vi "Main Read Processed Incoming Messages.vi"(8 "error in":errorcluster, 11 "internal data":T1={"J1939 XNET Settings"={"XNET Database"="", "XNET Cluster"="", "CAN port"="", "Baud rate [Bd]"=0, "J1939 Network Address"=0, "Name"=0, "Termination"=0}, "j1939 queues"={"Processed Outgoing"=refnum, "Process Outgoing"=refnum, "stop notifier"=refnum, "error queue"=refnum, "active dtc"=refnum, "processed inc"=refnum}, "fgv references"={"BAM Buffer"=refnum, "CM Buffer"=refnum, "CM Gen"=refnum, "BAM Gen"=refnum, "Address Claims"=refnum, "RQST"=refnum, "scaling lut"=refnum, "data lut"=refnum, "cyclic scheduler"=refnum}, "frame in"="", "frame out"="", "timing"={"tb to j1939 queue timeout"=100, "j1939 to tb queue timeout"=100, "dtc loop period (ms)"=100, "CAN in loop period (ms)"=100, "process incoming queue timeout (ms)"=100, "Outgoing Write Decimation"=0, "process outgoing loop rate (ms)"=0, "periodic outgoing queue timeout (ms)"=10, "CAN out queue timeout (ms)"=100}}) -> ()   [LabVIEW 2013, in "J1939.lvlib"]
uses:
  J1939.lvlib
  API Types/Internal Data.ctl
  API Types/XNET Settings.ctl
  API Types/Setup Information Cluster.ctl
  API Types/CAN Outgoing Message Cluster.ctl
  API Types/Convert DTCs Cluster.ctl
  <vilib>/xnet/xnet.llb/XNET Frame CAN.ctl
  <vilib>/xnet/xnet.llb/XNET Frame Type CAN.ctl
  TP/TP List References.ctl
  BAM/BAM Buffer Connections List_Ref.ctl
  Connection Mode/Connection Mode Generation Connection Ref.ctl
  BAM/BAM Generation Connections List_Ref.ctl
  LUTs/J1939 Address Table Reference.ctl
  RQST/RQST Lookup Table Reference.ctl
  LUTs/J1939 Conversion Lookup Table Reference.ctl
  LUTs/J1939 Data Lookup Table Reference.ctl
  LUTs/Cyclic Frame Scheduler Lut Reference.ctl
  Configuration/TypeDefs/timing configuration.ctl
  <vilib>/xnet/xnet.llb/XNET Convert (Frame Raw to Signal).vi
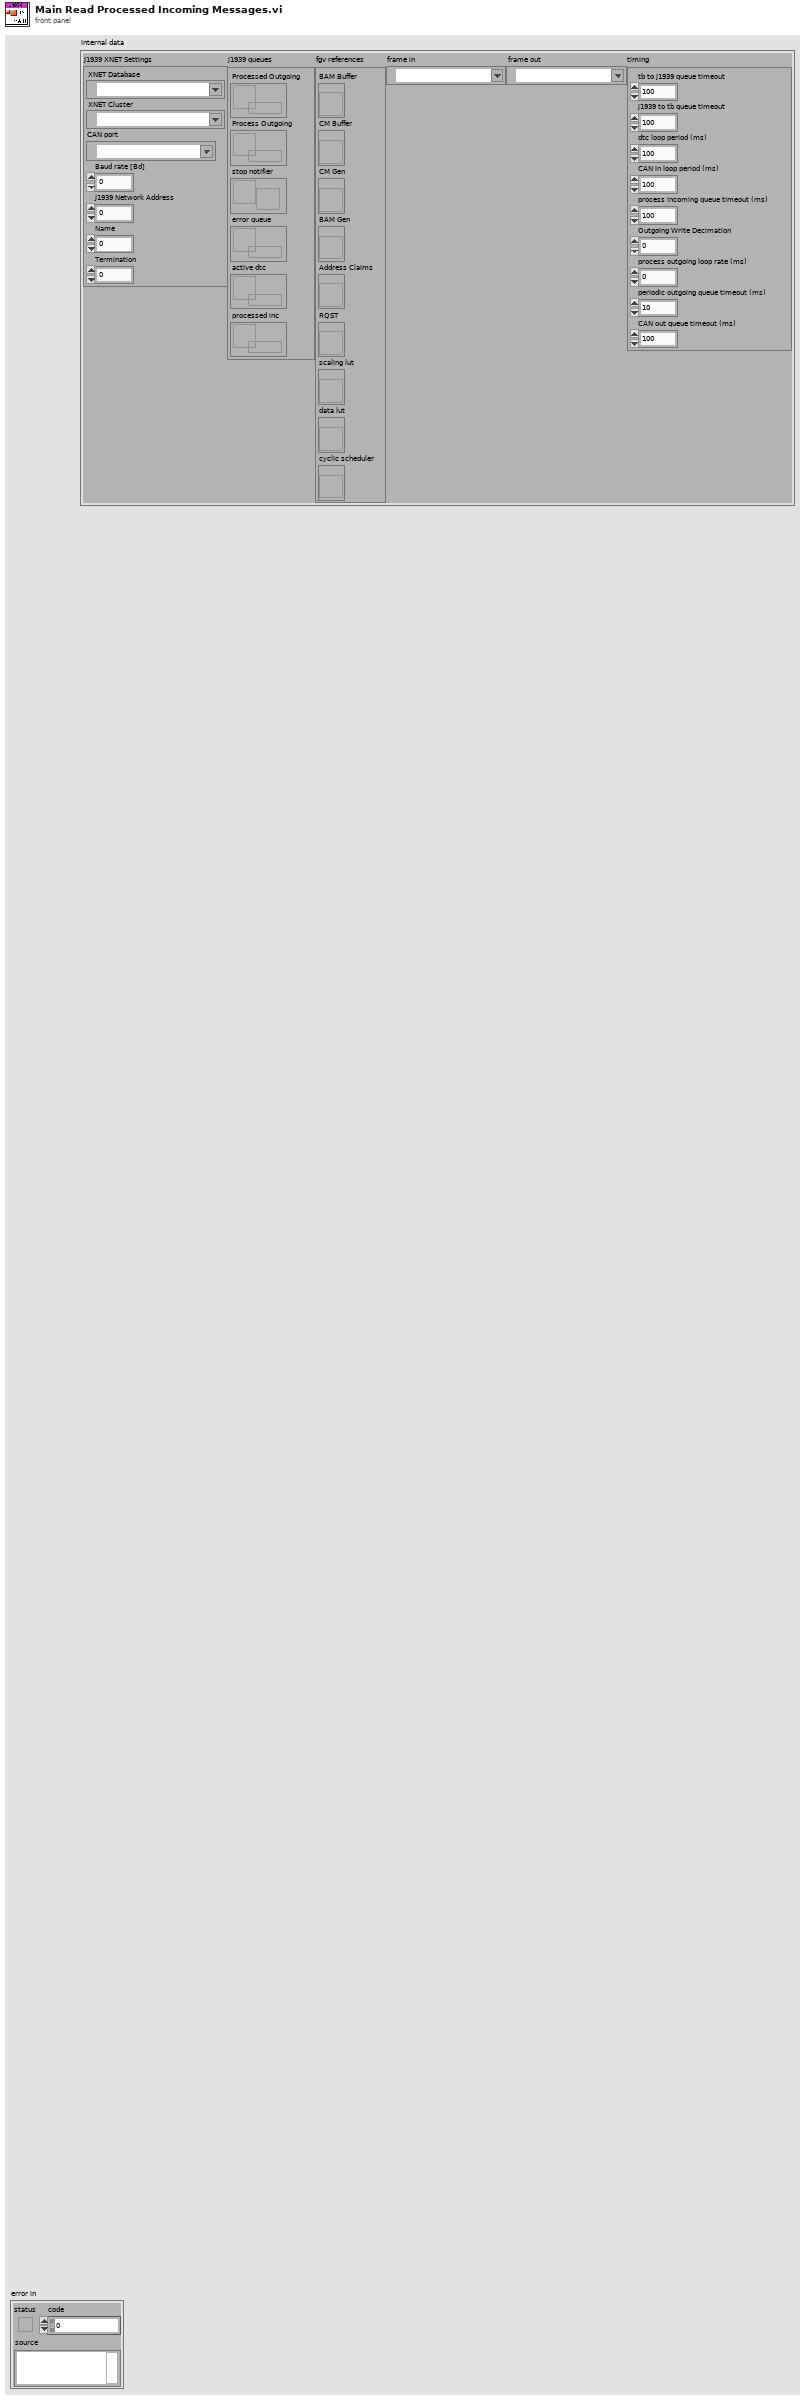
[diagram p1: front panel]
types:
  T1 = typedef "J1939.lvlib/Internal Data.ctl" = cluster{"J1939 XNET Settings":T2, "j1939 queues":T3, "fgv references":T4, "frame in":refnum<k21>, "frame out":refnum<k21>, "timing":T13}
  T2 = typedef "J1939.lvlib/XNET settings.ctl" = cluster{"XNET Database":refnum<k21>, "XNET Cluster":refnum<k21>, "CAN port":refnum<k21>, "Baud rate [Bd]":u32, "J1939 Network Address":u8, "Name":u64, "Termination":u32}
  T3 = typedef "J1939.lvlib/Setup Information Cluster.ctl" = cluster{"Processed Outgoing":refnum<queue>, "Process Outgoing":refnum<queue>, "stop notifier":refnum<notifier>, "error queue":refnum<queue>, "active dtc":refnum<queue>, "processed inc":refnum<queue>}
  T4 = typedef "J1939.lvlib/TP List References.ctl" = cluster{"BAM Buffer":T5, "CM Buffer":T5, "CM Gen":T6, "BAM Gen":T7, "Address Claims":T8, "RQST":T9, "scaling lut":T10, "data lut":T11, "cyclic scheduler":T12}
  T5 = typedef "J1939.lvlib/BAM Buffer Connections List_Ref.ctl" = refnum<vi>
  T6 = typedef "J1939.lvlib/Connection Mode Generation Connection Ref.ctl" = refnum<vi>
  T7 = typedef "J1939.lvlib/BAM Generation Connections List_Ref.ctl" = refnum<vi>
  T8 = typedef "J1939.lvlib/J1939 Address Table Reference.ctl" = refnum<vi>
  T9 = typedef "J1939.lvlib/RQST Lookup Table Reference.ctl" = refnum<vi>
  T10 = typedef "J1939.lvlib/J1939 Conversion Lookup Table Reference.ctl" = refnum<vi>
  T11 = typedef "J1939.lvlib/J1939 Data Lookup Table Reference.ctl" = refnum<vi>
  T12 = typedef "J1939.lvlib/cyclic frame scheduler lut reference.ctl" = refnum<vi>
  T13 = typedef "J1939.lvlib/timing configuration.ctl" = cluster{"tb to j1939 queue timeout":i32, "j1939 to tb queue timeout":i32, "dtc loop period (ms)":i32, "CAN in loop period (ms)":i32, "process incoming queue timeout (ms)":i32, "Outgoing Write Decimation":u32, "process outgoing loop rate (ms)":i32, "periodic outgoing queue timeout (ms)":i32, "CAN out queue timeout (ms)":i32}
  T14 = typedef "XNET Frame CAN.ctl" = cluster{"timestamp":timestamp, "payload":u8[], "identifier":u32, "type":T15, "extended?":bool, "echo?":bool}
  T15 = typedef "XNET Frame Type CAN.ctl" = u8
  T16 = typedef "J1939.lvlib/J1939 Conversion Lookup Table Parameters Cluster.ctl" = cluster{"Conversion":refnum<k21>, "Array Position":cluster{"Offset":u32, "Length":u32}, "Length":u32, "Conv ID":u32}
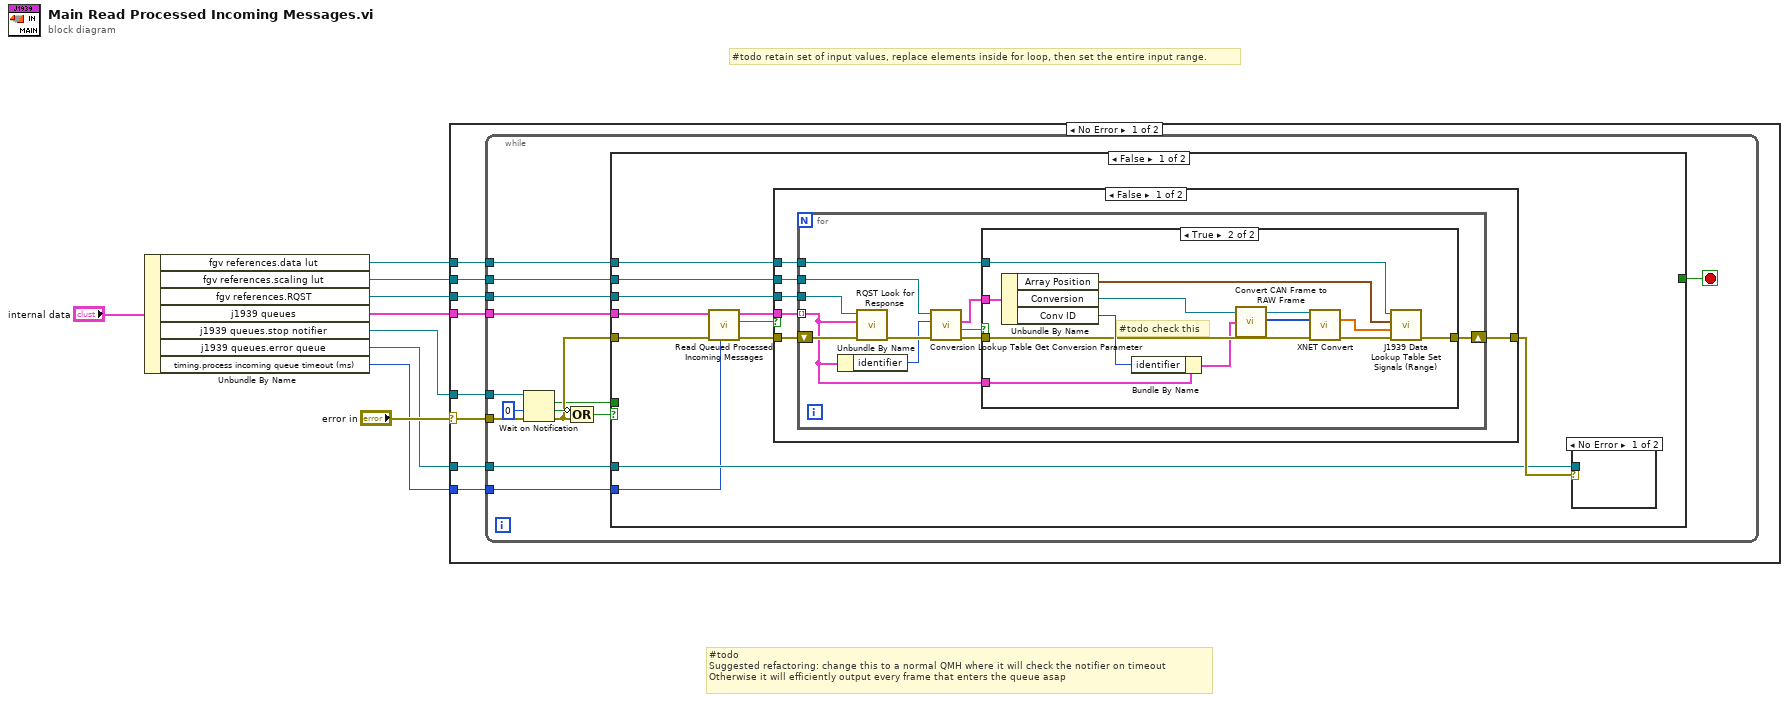
[diagram p0: block diagram]
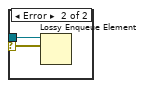
[diagram p2: hidden frame]
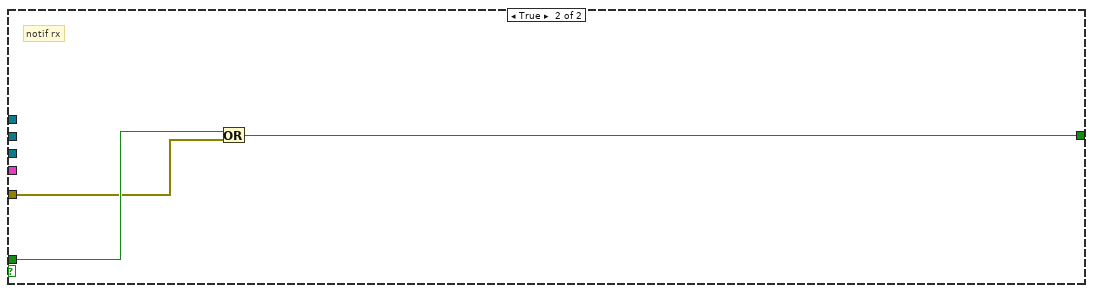
[diagram p5: hidden frame]
diagram:
  # "#todo retain set of input values, replace elements inside for loop, then set the entire input range."
  # "#todo\nSuggested refactoring: change this to a normal QMH where it will check the notifier on timeout\nOtherwise it will efficiently output every frame that enters the queue asap"
  n1 = Unbundle By Name("internal data") -> ("fgv references.data lut"=w4:T11, "fgv references.scaling lut"=w5:T10, "fgv references.RQST"=w6:T9, "j1939 queues"=w7:T3, "j1939 queues.stop notifier"=w3:refnum<notifier>, "j1939 queues.error queue"=w2:refnum<queue>, "timing.process incoming queue timeout (ms)"=w1:i32)
  n2 = case shown="No Error" "error in" {
    selector: "error in" -> [w17 _]
    tunnel: w3 -> [w16 _]
    tunnel: w7 -> [w15 _]
    tunnel: w6 -> [w14 _]
    tunnel: w5 -> [w13 _]
    tunnel: w4 -> [w12 _]
    tunnel: w2 -> [w11 _]
    tunnel: w1 -> [w10 _]
    frame No Error {
      n3 = while {
        tunnel: w16 -> [w19]
        tunnel: w17 -> [w31]
        tunnel: w15 -> [w25]
        tunnel: w14 -> [w24]
        tunnel: w13 -> [w23]
        tunnel: w12 -> [w22]
        tunnel: w11 -> [w20]
        tunnel: w10 -> [w18]
        stop <- w26 stop-if-true
        n4 = Wait on Notification(notifier=w19, timeout in ms (-1)=0, error in (no error)=w31) -> (notification=w27:bool, timed out?=w30:bool, error out=w28:errorcluster)  [unwired: 1 in, 1 out]
        n5 = Compound Arithmetic op=OR(invert w30, w28) -> (w29:bool)
        n6 = case shown="False" w29 {
          tunnel: w28 -> [w39 w76]
          tunnel: w27 -> [_ w78]
          tunnel: [_ w77] -> w26
          tunnel: w25 -> [w38 _]
          tunnel: w24 -> [w37 _]
          tunnel: w23 -> [w36 _]
          tunnel: w22 -> [w35 _]
          tunnel: w20 -> [w33 _]
          tunnel: w18 -> [w32 _]
          frame False {
            n7 = call "Read Queued Processed Incoming Messages.vi"("timeout in ms (-1)"=w32, "error in"=w39, "j1939 queues"=w38) -> ("error out"=w42:errorcluster, "timed out?"=w40:bool, "Frames"=w41:T14[])  [unwired: 6 in]
            n8 = case shown="False" w40 {
              tunnel: w36 -> [w50 _]
              tunnel: w35 -> [w49 _]
              tunnel: [w48 w75] -> w34
              tunnel: w37 -> [w47 _]
              tunnel: w42 -> [w46 w75]
              tunnel: w41 -> [w45 _]
              frame False {
                n9 = for {
                  tunnel: w50 -> [w61]
                  tunnel: w47 -> [w58]
                  tunnel: w45 -> [w56] mode=indexing
                  shift-right: [w59] -> w48
                  shift-left: w46 -> [w57]
                  tunnel: w49 -> [w60]
                  n10 = Unbundle By Name(w56) -> ("identifier"=w51:u32)
                  n11 = call "RQST Look for Response.vi"("error in (no error)"=w57, "CAN frame"=w56, "ref in"=w58) -> ("error out"=w52:errorcluster)  [unwired: 8 in]
                  n12 = call "Conversion Lookup Table Get Conversion Parameter.vi"("error in (no error)"=w52, "ID"=w51, "Ref in"=w61) -> ("error out"=w55:errorcluster, "Found?"=w53:bool, "Parameters"=w54:T16)  [unwired: 5 in, 1 out]
                  n13 = case shown="True" w53 {
                    tunnel: w55 -> [w62 w67]
                    tunnel: w54 -> [_ w74]
                    tunnel: w60 -> [_ w72]
                    tunnel: [w62 w66] -> w59
                    tunnel: w56 -> [_ w64]
                    frame False {
                    }
                    frame True {
                      # "#todo check this"
                      n14 = Unbundle By Name(w74) -> ("Array Position"=w71:cluster{"Offset":u32, "Length":u32}, "Conversion"=w70:refnum<k21>, "Conv ID"=w68:u32)
                      n15 = Bundle By Name(cluster=w64, "identifier"=w68) -> (w63:T14)
                      n16 = call "Convert CAN Frame to RAW Frame.vi"("CAN frame"=w63) -> ("RAW Data"=w65:u8[])  [unwired: 4 in]
                      n17 = call-poly <vilib>:"XNET Convert.vi"("session in"=w70, "frame data"=w65, "error in (no error)"=w67) -> ("signal data"=w69:dbl[], "error out"=w73:errorcluster)  [unwired: 10 in, 1 out]
                      n18 = call "J1939 Data Lookup Table Set Signals (Range).vi"("error in (no error)"=w73, "Signals"=w69, "Direct Access"=w71, "Ref in"=w72) -> ("error out"=w66:errorcluster)  [unwired: 6 in, 1 out]
                    }
                  }
                }
              }
              frame True {
              }
            }
            n19 = case shown="No Error" w34 {
              selector: w34 -> [_ w43]
              tunnel: w33 -> [_ w44]
              frame No Error {
              }
              frame Error {
                n20 = Lossy Enqueue Element(queue=w44, element=w43) -> ()  [unwired: 1 in, 4 out]
              }
            }
          }
          frame True {
            # "notif rx"
            n21 = Or(x=w78, y=w76) -> (x .or. y?=w77:bool)
          }
        }
      }
    }
    frame Error {
    }
  }
